vi "Set FPGA Properties.vi"(6 "FPGA Target":T1, 7 "Bitfile Path":path, 8 "error in (no error)":errorcluster, 9 "TargetClass":string, 10 "Signature":T2, 11 "Item Ref in":T3 format="%.0x") -> (0 "error out":errorcluster, 3 "Item Ref out":T3 format="%.0x")   [LabVIEW 2016, in "Scan Engine Custom Device.lvlib"]
uses:
  Scan Engine Custom Device.lvlib
  <vilib>/NI Veristand/Custom Device API/Custom Device API.lvlib
  <vilib>/NI Veristand/Custom Device API/Set Item Property (Path).vi
  Globals/Property Strings.vi
  Globals/String Constants.vi
  <vilib>/NI Veristand/Custom Device API/Set Item Property (String).vi
  <vilib>/NI Veristand/Custom Device API/Custom Device Supported Target.ctl
  <vilib>/NI Veristand/Custom Device API/Path Type.ctl
  <vilib>/NI Veristand/Custom Device API/Path Specification.ctl
  <vilib>/NI Veristand/Custom Device API/Custom Device File Dependency.ctl
  <vilib>/NI Veristand/Custom Device API/Set Item Property (U32).vi
  <vilib>/NI Veristand/Custom Device API/Custom Device Item Ref.ctl
  Type Defs/FPGA Target.ctl
  Type Defs/Bitfile Signature.ctl
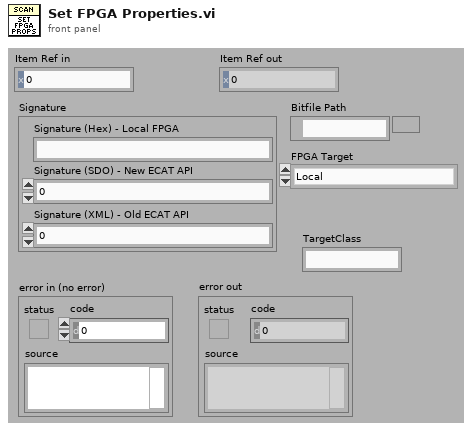
[diagram p1: front panel]
types:
  T1 = typedef "Scan Engine Custom Device.lvlib/FPGA Target.ctl" = enum16{"Local", "EtherCAT"}
  T2 = typedef "Scan Engine Custom Device.lvlib/Bitfile Signature.ctl" = cluster{"Signature (Hex) - Local FPGA":string, "Signature (SDO) - New ECAT API":u32, "Signature (XML) - Old ECAT API":u32}
  T3 = typedef "Custom Device API.lvlib/Custom Device Item Ref.ctl" = u64
  T4 = typedef "Custom Device API.lvlib/Custom Device Supported Target.ctl" = enum16{"All", "PharLap", "VxWorks", "Windows", "Linux_32_ARM", "Linux_x64", "PharLap & Windows", "PharLap & VxWorks", "VxWorks & Windows"}
  T5 = typedef "Custom Device API.lvlib/Custom Device File Dependency.ctl" = cluster{"Source":T6, "RT Destination":path, "ForceDownload?":bool, "SupportedTarget":T4, "Version":string}
  T6 = typedef "Custom Device API.lvlib/Path Specification.ctl" = cluster{"Path":path, "Type":T7}
  T7 = typedef "Custom Device API.lvlib/Path Type.ctl" = enum16{"Absolute", "To Base", "To Common Data Dir", "To Application Data Dir"}
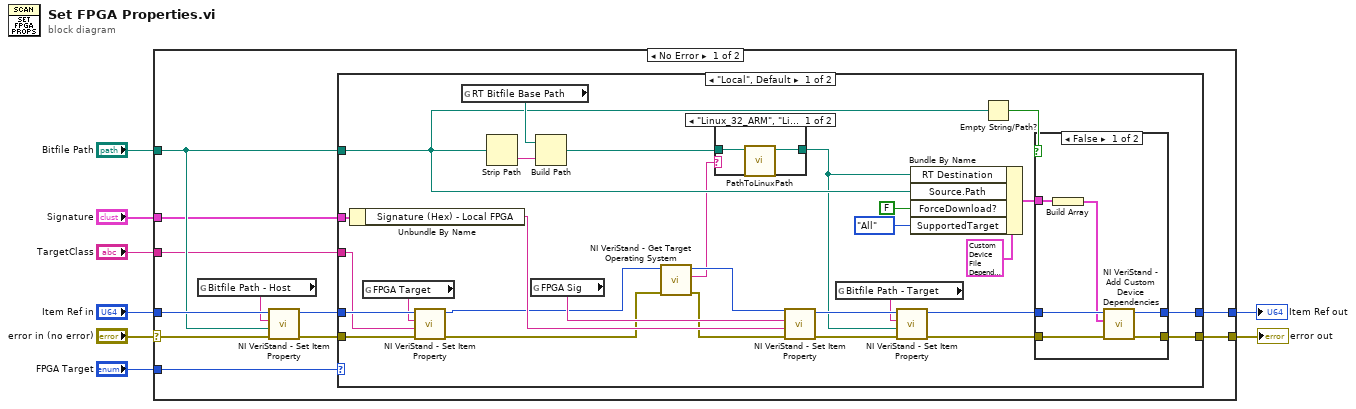
[diagram p0: block diagram]
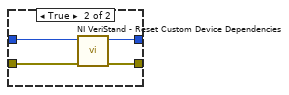
[diagram p3: hidden frame]
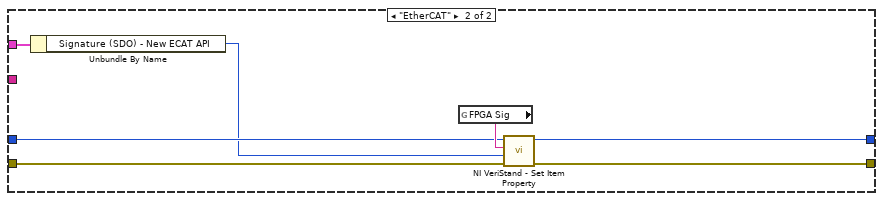
[diagram p4: hidden frame]
diagram:
  n1 = case shown="No Error" "error in (no error)" {
    selector: "error in (no error)" -> [w17 w70]
    tunnel: [w11 w70] -> w7
    tunnel: [w12 w69] -> w6
    tunnel: "Item Ref in" -> [w19 w69]
    tunnel: "Bitfile Path" -> [w16 _]
    tunnel: "FPGA Target" -> [w13 _]
    tunnel: "TargetClass" -> [w10 _]
    tunnel: "Signature" -> [w9 _]
    frame No Error {
      n2 = global read "Property Strings.vi" "Bitfile Path - Host"() -> (w18:string)
      n3 = call-poly <vilib>:"NI VeriStand - Set Item Property.vi"("error in (no error)"=w17, "Value"=w16, "Property Name"=w18, "Item Ref in"=w19) -> ("error out"=w14:errorcluster, "Item Ref out"=w15:T3)  [unwired: 5 in, 1 out]
      n4 = case shown="\"Local\", Default" w13 {
        tunnel: w16 -> [w29 _]
        tunnel: w15 -> [w46 w66]
        tunnel: w14 -> [w45 w67]
        tunnel: [w30 w63] -> w12
        tunnel: [w31 w62] -> w11
        tunnel: w10 -> [w42 _]
        tunnel: w9 -> [w44 w65]
        frame "Local", Default {
          n5 = Unbundle By Name(w44) -> ("Signature (Hex) - Local FPGA"=w40:string)
          n6 = global read "Property Strings.vi" "FPGA Target"() -> (w43:string)
          n7 = call-poly <vilib>:"NI VeriStand - Set Item Property.vi"("error in (no error)"=w45, "Value"=w42, "Property Name"=w43, "Item Ref in"=w46) -> ("error out"=w26:errorcluster, "Item Ref out"=w24:T3)  [unwired: 5 in, 1 out]
          n8 = global read "String Constants.vi" "RT Bitfile Base Path"() -> (w47:path)
          n9 = Strip Path(path=w29) -> (name=w48:string)  [unwired: 1 out]
          n10 = global read "Property Strings.vi" "FPGA Sig"() -> (w41:string)
          n11 = Build Path(base path=w47, name or relative path=w48) -> (appended path=w21:path)
          n12 = call "NI VeriStand - Get Target Operating System.vi"("error in (no error)"=w26, "Item Ref in"=w24) -> ("error out"=w25:errorcluster, "Operating System Name"=w22:string, "Item Ref out"=w23:T3)  [unwired: 7 in]
          n13 = case shown="\"Linux_32_ARM\", \"Linux_x64\"" w22 {
            tunnel: w21 -> [w50 w51]
            tunnel: [w49 w51] -> w20
            frame "Linux_32_ARM", "Linux_x64" {
              n14 = call "PathToLinuxPath.vi"("Path in"=w50) -> ("Path out"=w49:path)  [unwired: 10 in]
            }
            frame Default {
            }
          }
          n15 = call-poly <vilib>:"NI VeriStand - Set Item Property.vi"("error in (no error)"=w25, "Value"=w40, "Property Name"=w41, "Item Ref in"=w23) -> ("error out"=w39:errorcluster, "Item Ref out"=w38:T3)  [unwired: 5 in, 1 out]
          n16 = global read "Property Strings.vi" "Bitfile Path - Target"() -> (w27:string)
          n17 = call-poly <vilib>:"NI VeriStand - Set Item Property.vi"("error in (no error)"=w39, "Value"=w20, "Property Name"=w27, "Item Ref in"=w38) -> ("error out"=w36:errorcluster, "Item Ref out"=w37:T3)  [unwired: 5 in, 1 out]
          n18 = Bundle By Name(cluster=T5 {"Source"={"Path"=path "", "Type"=enum."Absolute"}, "RT Destination"=path "", "ForceDownload?"=FALSE, "SupportedTarget"=enum."PharLap", "Version"=""} ("Dependency"), "RT Destination"=w20, "Source.Path"=w29, "ForceDownload?"=FALSE, "SupportedTarget"=Custom_Device_Supported_Target."All") -> (w32:T5)
          n19 = Empty String/Path?(string/path=w29) -> (empty?=w28:bool)
          n20 = case shown="False" w28 {
            tunnel: w37 -> [w57 w59]
            tunnel: w36 -> [w56 w61]
            tunnel: w32 -> [w55 _]
            tunnel: [w52 w60] -> w31
            tunnel: [w53 w58] -> w30
            frame False {
              n21 = Build Array(w55) -> (w54:T5[])
              n22 = call <vilib>:"NI VeriStand - Add Custom Device Dependencies.vi"("error in (no error)"=w56, "Dependencies"=w54, "Device Ref in"=w57) -> ("error out"=w52:errorcluster, "Device Ref out"=w53:T3)  [unwired: 7 in]
            }
            frame True {
              n23 = call <vilib>:"NI VeriStand - Reset Custom Device Dependencies.vi"("error in (no error)"=w61, "Device Ref in"=w59) -> ("error out"=w60:errorcluster, "Device Ref out"=w58:T3)  [unwired: 8 in]
            }
          }
        }
        frame "EtherCAT" {
          n24 = Unbundle By Name(w65) -> ("Signature (SDO) - New ECAT API"=w64:u32)
          n25 = global read "Property Strings.vi" "FPGA Sig"() -> (w68:string)
          n26 = call-poly <vilib>:"NI VeriStand - Set Item Property.vi"("error in (no error)"=w67, "Value"=w64, "Property Name"=w68, "Item Ref in"=w66) -> ("error out"=w62:errorcluster, "Item Ref out"=w63:T3)  [unwired: 5 in, 1 out]
        }
      }
    }
    frame Error {
    }
  }
  "Item Ref out" <- w6
  "error out" <- w7
